vi "Table, Fill Column Value, String.vi"(6 "column (0)":i32, 8 "error in":errorcluster, 10 "Value (\"\")":string, 11 "Tbl Refnum":refnum<vi>) -> (0 "error out":errorcluster, 3 "Tbl Refnum out":refnum<vi>)   [LabVIEW 2010]
doc: "Converts one row from a Test Criteria Table to a TestStand Result cluster."
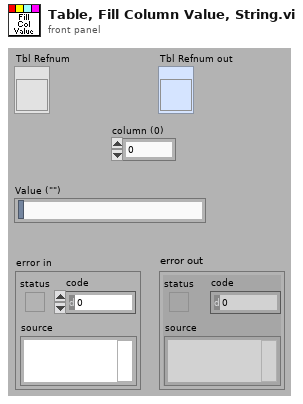
[diagram p1: front panel]
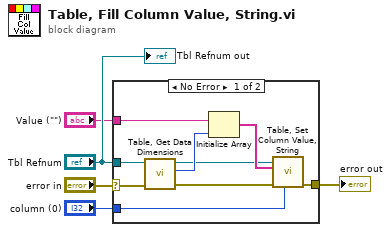
[diagram p0: block diagram]
diagram:
  n1 = case shown="No Error" "error in" {
    selector: "error in" -> [w14 w15]
    tunnel: "Tbl Refnum" -> [w8 _]
    tunnel: [w12 w15] -> w5
    tunnel: "column (0)" -> [w6 _]
    tunnel: "Value (\"\")" -> [w10 _]
    frame No Error {
      n2 = call "Table, Get Data Dimensions.vi"("error in"=w14, "Tbl Refnum"=w8) -> ("error out"=w13:errorcluster, "row_n"=w11:i32, "Tbl Refnum out"=w7:refnum<vi>)  [unwired: 6 in, 1 out]
      n3 = Initialize Array(w10, w11) -> (w9:string[])
      n4 = call "Table, Set Column Value, String.vi"("column (0)"=w6, "error in"=w13, "Value"=w9, "Tbl Refnum"=w7) -> ("error out"=w12:errorcluster)  [unwired: 5 in, 2 out]
    }
    frame Error {
    }
  }
  "error out" <- w5
  "Tbl Refnum out" <- "Tbl Refnum"
